vi "CRYTree Manipulate Asist.vi"(7 "sAction":string, 9 "sNewTags":string[](array[string]), 10 "sOrgTags":string[](array[string]), 11 "Tree in":refnum<vi>) -> (0 "bResult Out":bool, 1 "sData Out":string[](array[string]), 3 "Tree Out":refnum<vi>)   [LabVIEW 2013]
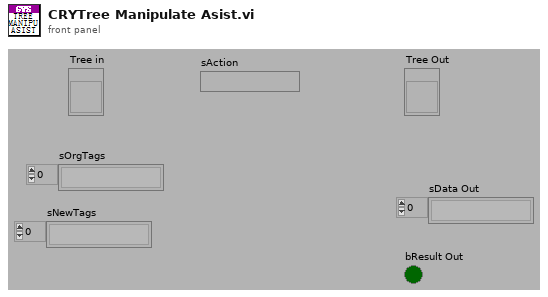
[diagram p1: front panel]
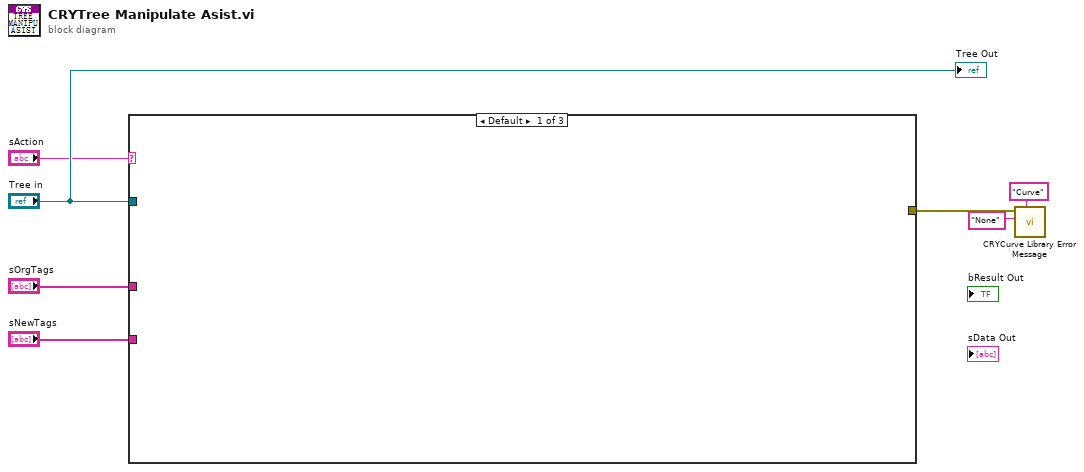
[diagram p0: block diagram]
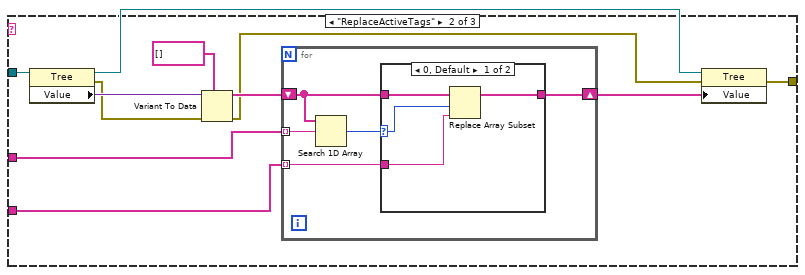
[diagram p2: hidden frame]
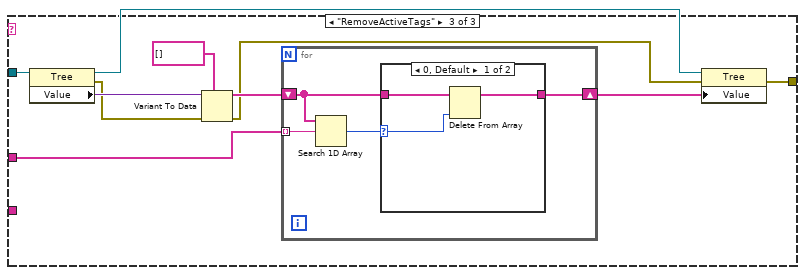
[diagram p4: hidden frame]
diagram:
  n1 = case shown="Default" "sAction" {
    tunnel: "Tree in" -> [_ w18 w38]
    tunnel: "sOrgTags" -> [_ w17 w37]
    tunnel: "sNewTags" -> [_ w16 _]
    tunnel: [_ w10 w31] -> w1
    frame Default {
    }
    frame "ReplaceActiveTags" {
      n2 = property class="Tree"(reference=w18) -> (reference out=w11:refnum<vi>, error out=w9:errorcluster, "Value"=w15:variant)  [unwired: 1 in]
      n3 = Variant To Data(error in=w9, type=string[] [] ("Selected Rows"), Variant=w15) -> (data=w13:string[], error out=w8:errorcluster)
      n4 = for {
        tunnel: w17 -> [w20] mode=indexing
        shift-right: [w21] -> w12
        shift-left: w13 -> [w22]
        tunnel: w16 -> [w19] mode=indexing
        n5 = Search 1D Array(1D array=w22, element=w20) -> (index of element=w23:i32)  [unwired: 1 in]
        n6 = case shown="0, Default" w23 {
          selector: w23 -> [w24 _]
          tunnel: w22 -> [w27 w28]
          tunnel: [w26 w28] -> w21
          tunnel: w19 -> [w25 _]
          frame 0, Default {
            n7 = Replace Array Subset(array=w27, new element=w25, index=w24) -> (w26:string[])
          }
          frame -1 {
          }
        }
      }
      n8 = property class="Tree"(reference=w11, error in=w8, "Value"=w12) -> (error out=w10:errorcluster)  [unwired: 1 out]
    }
    frame "RemoveActiveTags" {
      n9 = property class="Tree"(reference=w38) -> (reference out=w32:refnum<vi>, error out=w30:errorcluster, "Value"=w36:variant)  [unwired: 1 in]
      n10 = Variant To Data(error in=w30, type=string[] [] ("Selected Rows"), Variant=w36) -> (data=w34:string[], error out=w29:errorcluster)
      n11 = for {
        tunnel: w37 -> [w39] mode=indexing
        shift-right: [w40] -> w33
        shift-left: w34 -> [w41]
        n12 = Search 1D Array(1D array=w41, element=w39) -> (index of element=w42:i32)  [unwired: 1 in]
        n13 = case shown="0, Default" w42 {
          selector: w42 -> [w43 _]
          tunnel: w41 -> [w45 w46]
          tunnel: [w44 w46] -> w40
          frame 0, Default {
            n14 = Delete From Array(array=w45, index=w43) -> (array with subset deleted=w44:string[])  [unwired: 1 in, 1 out]
          }
          frame -1 {
          }
        }
      }
      n15 = property class="Tree"(reference=w32, error in=w29, "Value"=w33) -> (error out=w31:errorcluster)  [unwired: 1 out]
    }
  }
  n16 = call "CRYCurve Library Error Message.vi"("sAction"="Curve", "sOption"="None", "error IO"=w1) -> ()  [unwired: 9 in]
  "Tree Out" <- "Tree in"
